vi "Single Control Loop.vi"() -> ()   [LabVIEW 2011]
uses:
  BotCommands.ctl
  vi/clearpath_interface.lvlib
panel:
  in  "VISA resource name":refnum<visa-resource-name>="ASRL1::INSTR"
  in  "Translational 2":dbl(slide) scale=-0.1..0.1
  in  "Translational":dbl(slide) scale=-0.1..0.1
  in  "error IO":errorcluster
  out "Left":dbl
  out "Right":dbl
  out "Msgs (total)":u32
  out "Network Timeout?":bool=TRUE
  out "Rotation":dbl(knob) scale=1.0..-1.0
  out "Speed":dbl(knob) scale=-1.0..1.0
  in  "Stop Interface":bool
  in  "Stop Motors?":bool
  in  "stop":bool
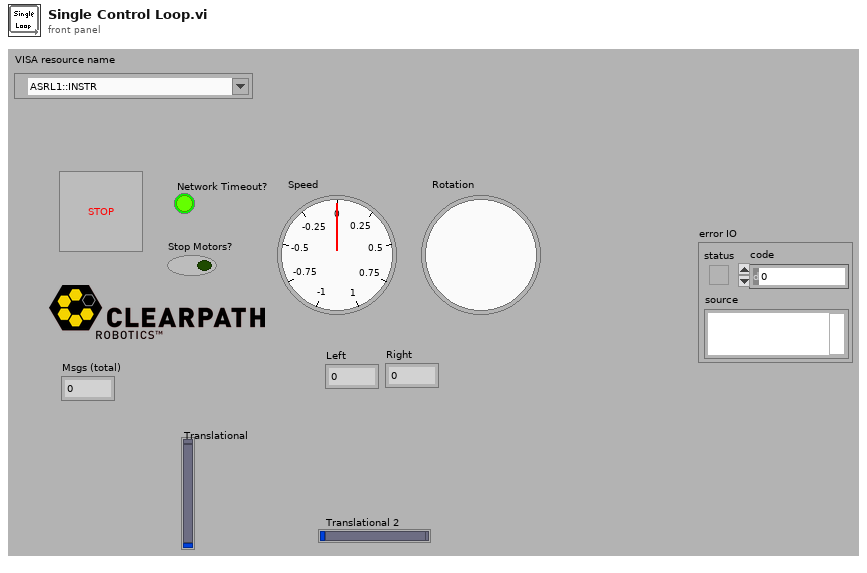
[diagram p1: front panel]
types:
  T1 = cluster{"Xmit Queue":refnum<queue>, "Data Queue":refnum<queue>, "VISA resource name out":refnum<visa-resource-name>, "error out":errorcluster, "Message Data Cluster":cluster{"\nChar Idx":u8, "Num. Char Rem":u8, "Write Index":u8, "Read Index":u8, "Message Data Buffer":u8[][]}}
  T2 = typedef "BotCommands.ctl" = cluster{"Translational":dbl, "Rotational":dbl}
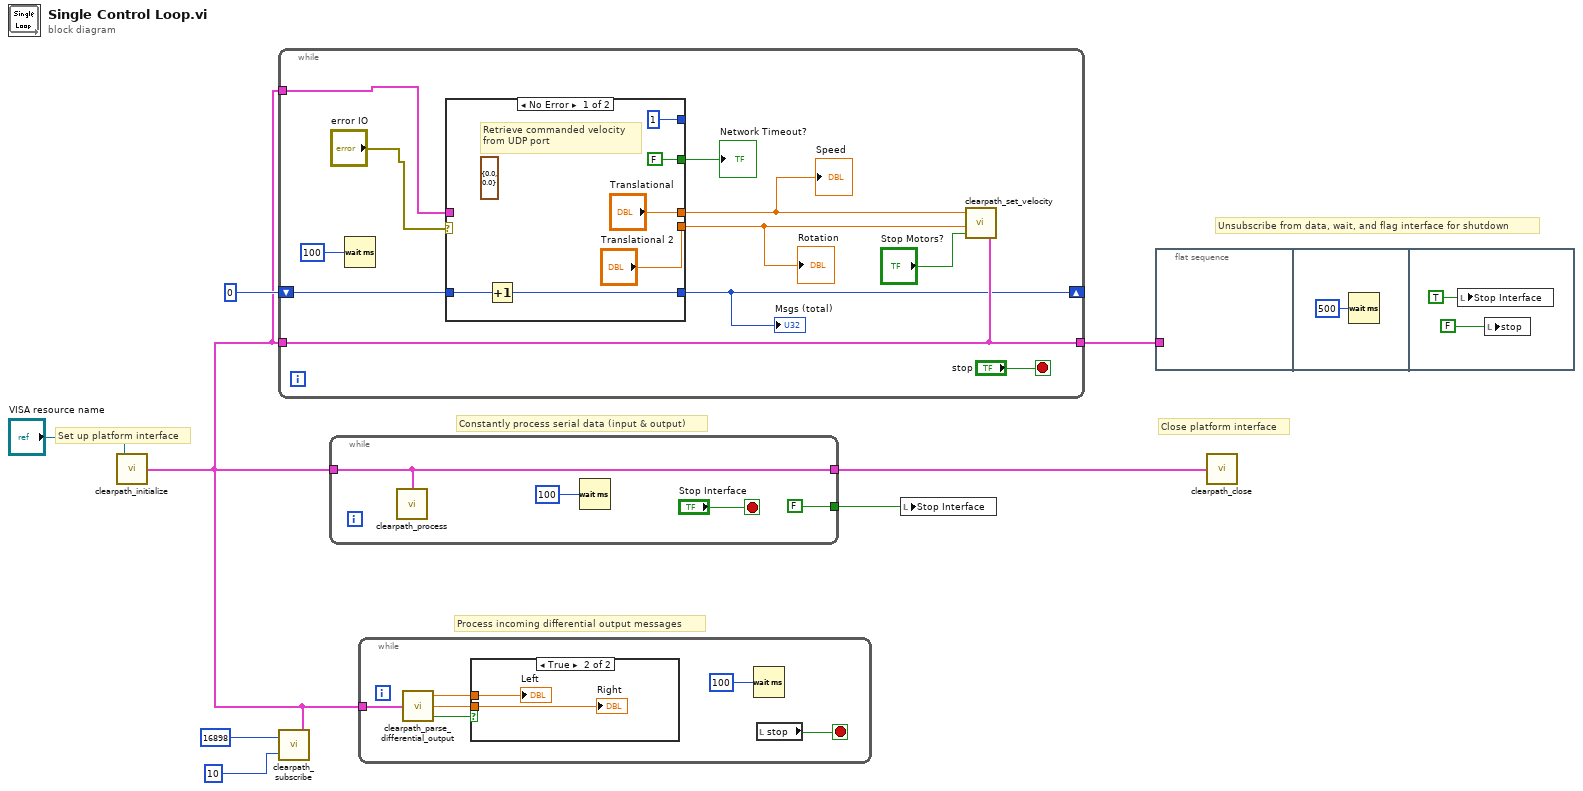
[diagram p0: block diagram]
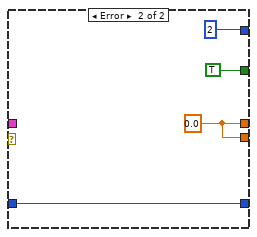
[diagram p3: hidden frame]
diagram:
  # "Process incoming differential output messages"
  # "Constantly process serial data (input & output)"
  # "Close platform interface"
  # "Unsubscribe from data, wait, and flag interface for shutdown"
  # "Set up platform interface"
  n1 = call "clearpath_initialize.vi"("VISA resource name"="VISA resource name") -> ("ClearpathComm"=w2:T1)  [unwired: 1 in]
  n2 = while {
    tunnel: w2 -> [w15]
    tunnel: [w15] -> w8
    shift-right: [w12] -> _
    shift-left: 0 -> [w13]
    tunnel: w2 -> [w9]
    stop <- "stop" stop-if-true
    n3 = Wait (ms)(milliseconds to wait=u32 100) -> ()  [unwired: 1 out]
    n4 = case shown="No Error" "error IO" {
      tunnel: ["Translational" w29] -> w18
      tunnel: ["Translational 2" w29] -> w17
      tunnel: w9 -> [_ _]
      tunnel: [FALSE TRUE] -> w16
      tunnel: w13 -> [w24 w27]
      tunnel: [w23 w27] -> w12
      tunnel: [1 2] -> _
      frame No Error {
        (unwired) T2 {"Translational"=0.0, "Rotational"=0.0} ("BotCommands")
        # "Retrieve commanded velocity\nfrom UDP port"
        n5 = Increment(x=w24) -> (x+1=w23:i32)
      }
      frame Error {
        w29 = 0.0 ("Translational")
      }
    }
    "Speed" <- w18
    "Rotation" <- w17
    "Network Timeout?" <- w16
    "Msgs (total)" <- w12
    n6 = call "clearpath_set_velocity.vi"("ClearpathComm"=w15, "Zero Speeds"="Stop Motors?", "Rotational Speed"=w17, "Translational Speed"=w18) -> ()
  }
  n7 = call "clearpath_subscribe.vi"("ClearpathComm"=w2, "Frequency"=10, "Message Type"=16898) -> ()
  n8 = while {
    tunnel: w2 -> [w31]
    tunnel: [w31] -> w6
    tunnel: [FALSE ("Stop Interface")] -> w5
    stop <- "Stop Interface" stop-if-true
    n9 = call "clearpath_process.vi"("ClearpathComm"=w31) -> ()
    n10 = Wait (ms)(milliseconds to wait=u32 100) -> ()  [unwired: 1 out]
  }
  n11 = while {
    tunnel: w2 -> [w36]
    stop <- w35 stop-if-true
    n12 = call "clearpath_parse_differential_output.vi"("ClearpathComm"=w36) -> ("Data Valid?"=w37:bool, "Right Output"=w38:dbl, "Left Output"=w39:dbl)
    n13 = case shown="True" w37 {
      tunnel: w39 -> [_ w41]
      tunnel: w38 -> [_ w40]
      frame False {
      }
      frame True {
        "Left" <- w41
        "Right" <- w40
      }
    }
    n14 = Wait (ms)(milliseconds to wait=u32 100) -> ()  [unwired: 1 out]
    n15 = local read "stop"() -> (w35:bool)
  }
  n16 = local write "Stop Interface"(w5) -> ()
  n17 = flat-sequence {
    tunnel: w8 -> [_]
    frame #0 {
    }
    frame #1 {
      n18 = Wait (ms)(milliseconds to wait=u32 500) -> ()  [unwired: 1 out]
    }
    frame #2 {
      n19 = local write "Stop Interface"(TRUE ("Stop Interface")) -> ()
      n20 = local write "stop"(FALSE ("stop")) -> ()
    }
  }
  n21 = call "clearpath_close.vi"("ClearpathComm"=w6) -> ()
